vi "mainActivity__启动所需要打开的所有vi.vi"() -> (0 "所需要打开的所有vi参数":cluster{"message":string, "data":variant}[](array[cluster]))   [LabVIEW 2014]
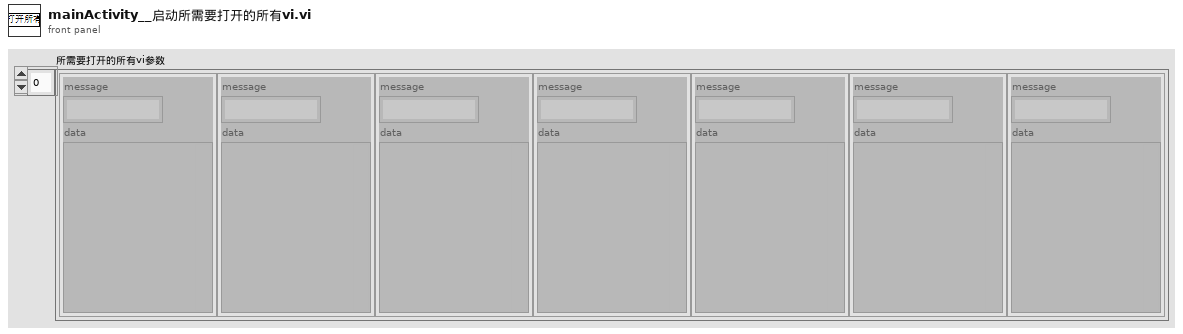
[diagram p1: front panel]
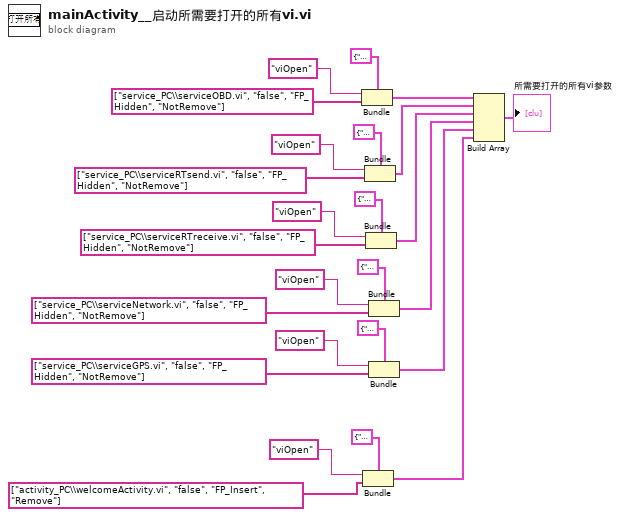
[diagram p0: block diagram]
diagram:
  n1 = Bundle(cluster=cluster{"message":string, "data":variant} {"message"="", "data"=variant} ("元素"), "message"="viOpen", "data"=string[] ["service_PC\\serviceOBD.vi", "false", "FP_Hidden", "NotRemove"]) -> (w10:cluster{"message":string, "data":variant})
  n2 = Bundle(cluster=cluster{"message":string, "data":variant} {"message"="", "data"=variant} ("元素"), "message"="viOpen", "data"=string[] ["activity_PC\\welcomeActivity.vi", "false", "FP_Insert", "Remove"]) -> (w6:cluster{"message":string, "data":variant})
  n3 = Bundle(cluster=cluster{"message":string, "data":variant} {"message"="", "data"=variant} ("元素"), "message"="viOpen", "data"=string[] ["service_PC\\serviceRTsend.vi", "false", "FP_Hidden", "NotRemove"]) -> (w9:cluster{"message":string, "data":variant})
  n4 = Bundle(cluster=cluster{"message":string, "data":variant} {"message"="", "data"=variant} ("元素"), "message"="viOpen", "data"=string[] ["service_PC\\serviceRTreceive.vi", "false", "FP_Hidden", "NotRemove"]) -> (w8:cluster{"message":string, "data":variant})
  n5 = Bundle(cluster=cluster{"message":string, "data":variant} {"message"="", "data"=variant} ("元素"), "message"="viOpen", "data"=string[] ["service_PC\\serviceNetwork.vi", "false", "FP_Hidden", "NotRemove"]) -> (w7:cluster{"message":string, "data":variant})
  n6 = Bundle(cluster=cluster{"message":string, "data":variant} {"message"="", "data"=variant} ("元素"), "message"="viOpen", "data"=string[] ["service_PC\\serviceGPS.vi", "false", "FP_Hidden", "NotRemove"]) -> (w1:cluster{"message":string, "data":variant})
  n7 = Build Array(w10, w9, w8, w7, w1, w6) -> (→"所需要打开的所有vi参数":cluster{"message":string, "data":variant}[])
